vi "turn left (SubVI).vi"(6 "Angle":dbl, 8 "error in (no error)":errorcluster, 11 "KNR in":T1) -> (0 "error out":errorcluster, 3 "KNR out":T1)   [LabVIEW 2013]
uses:
  <userlib>/KNR OS 3.0 LabVIEW Toolkit/Type Definition/KNR3 Reference.ctl
  <userlib>/_FPGA Interface Advanced Tools/FPGA Interface Base/FPGA Interface Base.lvclass
  <userlib>/KNR OS 3.0 LabVIEW Toolkit/Type Definition/Resource.ctl
panel:
  in  "STOP":bool
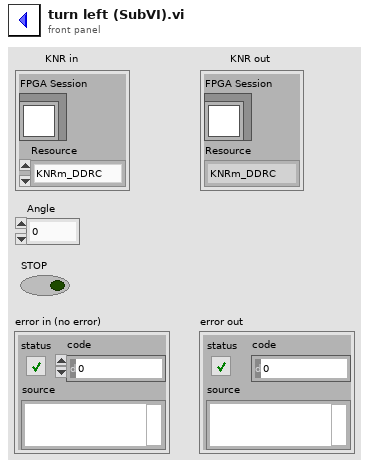
[diagram p1: front panel]
types:
  T1 = typedef "KNR3 Reference.ctl" = cluster{"FPGA Session":refnum<class "FPGA Interface Base.lvclass">, "Resource":T2}
  T2 = typedef "Resource.ctl" = enum16{"KNRm_DDRC", "KNRm_DDDD", "KNRm_DDDR", "KNRm_DDDC", "KNR"}
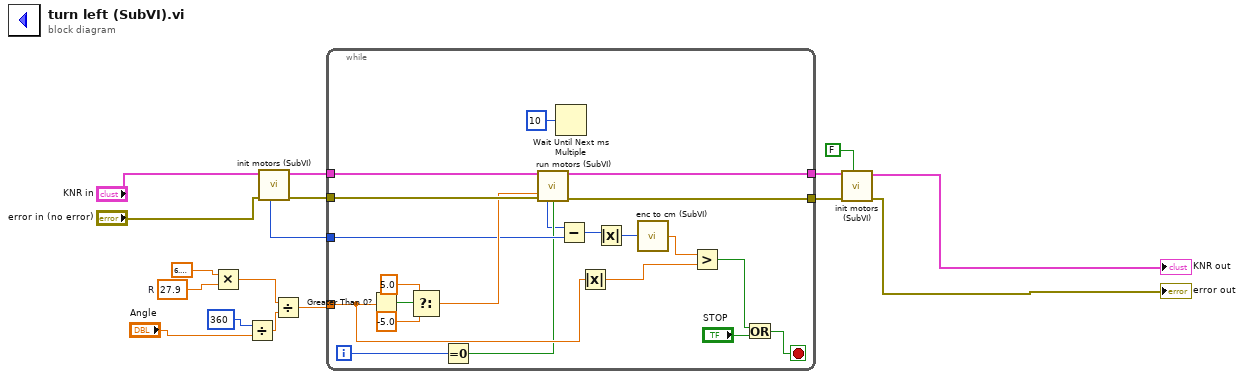
[diagram p0: block diagram]
diagram:
  w5 = 27.9  # R
  n1 = Multiply(x=6.283185307179586, y=w5) -> (x*y=w4:dbl)
  n2 = Divide(x=360, y="Angle") -> (x/y=w3:dbl)
  n3 = call "init motors (SubVI).vi"("error in (no error)"="error in (no error)", "KNR in"="KNR in") -> ("error out"=w16:errorcluster, "KNR out"=w17:T1, "Position_2"=w8:i32)  [unwired: 6 in, 1 out]
  n4 = Divide(x=w4, y=w3) -> (x/y=w2:dbl)
  n5 = while {
    tunnel: w17 -> [w38]
    tunnel: w16 -> [w37]
    tunnel: w2 -> [w30]
    tunnel: [w32] -> w14
    tunnel: [w31] -> w15
    tunnel: w8 -> [w29]
    i -> [w23]
    stop <- w26 stop-if-true
    n6 = Greater Than 0?(x=w30) -> (x > 0?=w36:bool)
    n7 = Select(t=5.0, s=w36, f=-5.0) -> (s? t:f=w33:dbl)
    n8 = Equal To 0?(x=w23) -> (x = 0?=w22:bool)
    n9 = call "run motors (SubVI).vi"("KNR in"=w38, "speed_2"=w33, "error in (no error)"=w37, "reinitialize? (F)"=w22) -> ("KNR out 2"=w32:T1, "Position_2"=w21:i32, "error out"=w31:errorcluster)  [unwired: 8 in, 1 out]
    n10 = Wait Until Next ms Multiple(millisecond multiple=u32 10) -> ()  [unwired: 1 out]
    n11 = Subtract(x=w21, y=w29) -> (x-y=w28:i32)
    n12 = Absolute Value(x=w30) -> (abs(x)=w27:dbl)
    n13 = Absolute Value(x=w28) -> (abs(x)=w19:i32)
    n14 = call "enc to cm (SubVI).vi"("E"=w19) -> ("CM"=w18:dbl)
    n15 = Greater?(x=w18, y=w27) -> (0:w25:bool)
    n16 = Or(x=w25, y="STOP") -> (x .or. y?=w26:bool)
  }
  n17 = call "init motors (SubVI).vi"("Enable Motor(T)"=FALSE, "error in (no error)"=w15, "KNR in"=w14) -> ("error out"=→"error out":errorcluster, "KNR out"=→"KNR out":T1)  [unwired: 5 in, 2 out]
